vi "Stop Core.vi"(10 "final error code":i32, 11 "Aumentar_contador in":refnum<class "Aumentar_contador.lvclass">) -> (3 "Aumentar_contador out":refnum<class "Aumentar_contador.lvclass">)   [LabVIEW 2019, in "Aumentar_contador.lvlib" / "Aumentar_contador.lvclass"]
doc: "(<B>Filename</B>: Actor Framework.lvlib:Actor.lvclass:Stop Core.vi)\n\nDefines what the actor does before it stops. Use the <B>final error code</B> input to determine whether the actor shut down in response to an error.\n\nBy default, this method passes the Stop message along to all auto-stop nested actors. A descendant class may override this method to define additional behavior, such as shutting down any processes the actor initiated in its override of the Actor Core method."
uses:
  Aumentar_contador.lvclass
  <vilib>/ActorFramework/Actor/Actor.lvclass
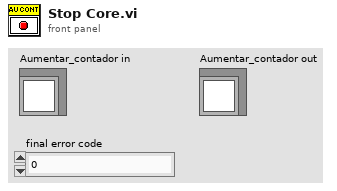
[diagram p1: front panel]
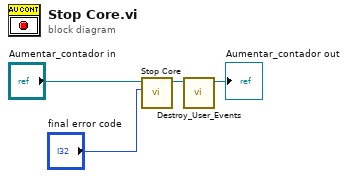
[diagram p0: block diagram]
diagram:
  n1 = call-parent "Stop Core.vi"("final error code"="final error code", "Actor in"="Aumentar_contador in") -> ("Actor out"=w2:refnum<class "Aumentar_contador.lvclass">)  [unwired: 9 in]
  n2 = call "Destroy_User_Events.vi"("Aumentar_contador in"=w2) -> ("Aumentar_contador out"=→"Aumentar_contador out":refnum<class "Aumentar_contador.lvclass">)  [unwired: 9 in, 1 out]
